vi "InstructEnqueue.vi"(8 "error in (no error)":errorcluster, 9 "Subsystem":T1=enum."ClimbWeight", 10 "Variant":variant, 11 "Queue":refnum<queue>) -> (0 "error out":errorcluster)   [LabVIEW 2013]
uses:
  QueueInstruction.ctl
  SubsystemEnum.ctl
  ActionEnum.ctl
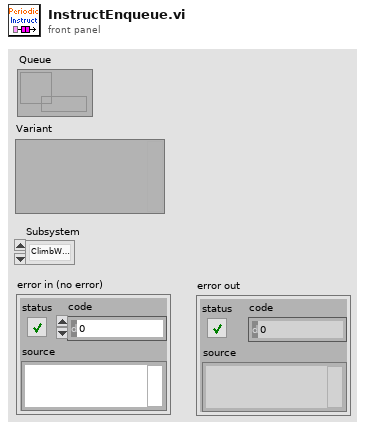
[diagram p1: front panel]
types:
  T1 = typedef "SubsystemEnum.ctl" = enum16{"TankDrive", "FirePneumatic", "Climber", "ClimbWeight", "ShooterAngle"}
  T2 = typedef "ActionEnum.ctl" = enum16{"Init", "SetValue"}
  T3 = typedef "QueueInstruction.ctl" = cluster{"Data":variant, "Subsystem":T1, "Action":T2}
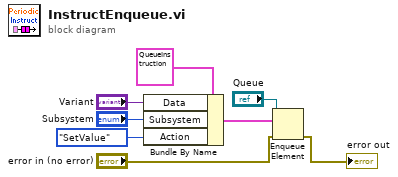
[diagram p0: block diagram]
diagram:
  n1 = Bundle By Name(cluster=T3 {"Data"=variant, "Subsystem"=enum."TankDrive", "Action"=enum."Init"} ("QueueInstruction"), "Data"="Variant", "Subsystem"="Subsystem", "Action"=ActionEnum."SetValue") -> (w6:T3)
  n2 = Enqueue Element(queue="Queue", element=w6, error in (no error)="error in (no error)") -> (error out=→"error out":errorcluster)  [unwired: 1 in, 2 out]
